vi "RecordAudioRoutedMessageName.vi"() -> (1 "message name":string)   [LabVIEW 2017, in "EmsaAcquisition.lvlib"]
uses:
  <vilib>/addons/InsightCM/Devices/Shared/Emsa/EmsaAcquisition/EmsaAcquisition.lvlib
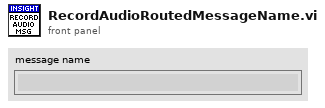
[diagram p1: front panel]
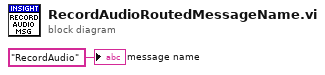
[diagram p0: block diagram]
diagram:
  "message name" <- "RecordAudio" ("ProcessName")
